vi "Basic Serial Write and Read Modified.vi"(0 "VISA resource name":refnum<visa-resource-name>="COM1", 1 "baud rate":u32=9600, 2 "data bits":u16=8 min=5 max=8 step=1, 3 "parity":u16(ring) items=["None", "Odd", "Even", "Mark", "Space"], 4 "stop bits":u16(ring)=10 items=["1.0"=10, "1.5"=15, "2.0"=20], 6 "read":bool=TRUE, 7 "flow control":u16(ring) items=["None"=0, "XON/XOFF"=1, "RTS/CTS"=2, "DTR/DSR"=4]) -> (9 "read string":string, 10 "bytes read":u32)   [LabVIEW 2016]
doc: "The Basic Serial Read and Write example performs a Serial Port Read, a Serial Port Write, or a combination of these actions. The user selects the actions (read or write) on the front panel. If both are selected, the VI will write the data first, read data, and then close the VISA session that is opened to the port. This VI will wait until the specified number of bytes is received at the port or until a termination character is read.\n\nINSTRUCTIONS:\n1) Select the serial resource and configuration parameters (baud rate, data bits, parity, stop bits, flow control).\n2) Select the operations to be performed. \n3) Connect the serial port to your device. If no device is available, perform a loopback test by doing one of the following. Short pins 2 and 3 on a RS-232 cable or short pin 4 to pin 8 and pin 5 to pin 9 on a RS-485/422 cable. \n4) Run the VI to see the data read. (The \"read string\" will match the \"string to write\" if a loopback test was performed.)\n\nNote: The parameters set for the serial port must match the parameters of the connected instrument or device. In this example, the bytes to read parameter specifies the number of bytes that the serial port reads. If there were more bytes at the port than the number specified in bytes to read, those bytes would not be read. Also, if you specify to read more bytes than the number of bytes actually read, you might receive a timeout error message.\n\nOn the block diagram, the Configure Serial Port VI sets the configuration parameters. The front panel displays the controls used to configure the basic parameters, such as baud rate, data bits, and parity. Constants configure the other parameters the user probably does not need set. After the VISA Configure Serial Port VI opens the VISA session and configures the port, the VI passes the VISA resource name to other VIs that perform operations on that VISA resource. The VISA Write function sends a command to the serial device and the VISA Read function returns data based on the command. The VISA Close function then closes the reference to the serial device. It is important to close the reference; otherwise communication through with that port through protocols other than VISA might not be possible."
uses:
  <vilib>/Instr/_visa.llb/VISA Configure Serial Port (Instr).vi
panel:
  in  "Stop":bool
  in  "Enable Termination\n Charactetr":bool
  in  "delay before read (ms)":u32=500
  # "On Windows/Linux, consider using the Instrument Driver Finder (Help>>Find Instrument Drivers) to search for an instrument driver for your instrument."
  # "Select the serial resource and the operations (Read, Write, or both) to be performed.  If both are selected, the VI will write the data first, read data and then close the VISA session that is opened to the port.  This VI will wait until the specified number of bytes is received at the port or until a termination character is read."
  # "For additional information select File >> VI Properties >> Documentation"
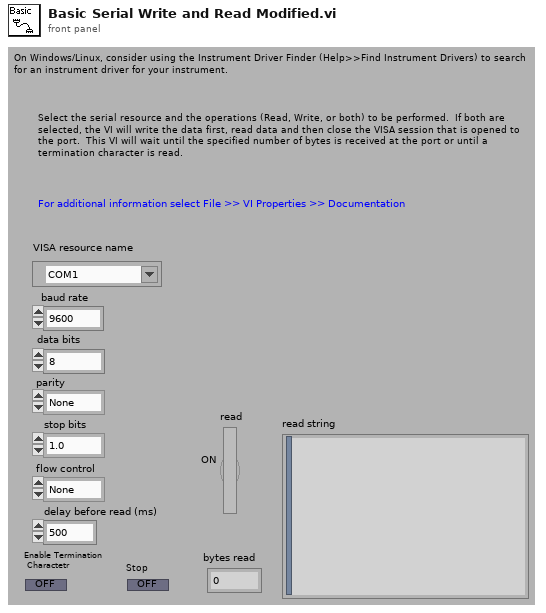
[diagram p1: front panel]
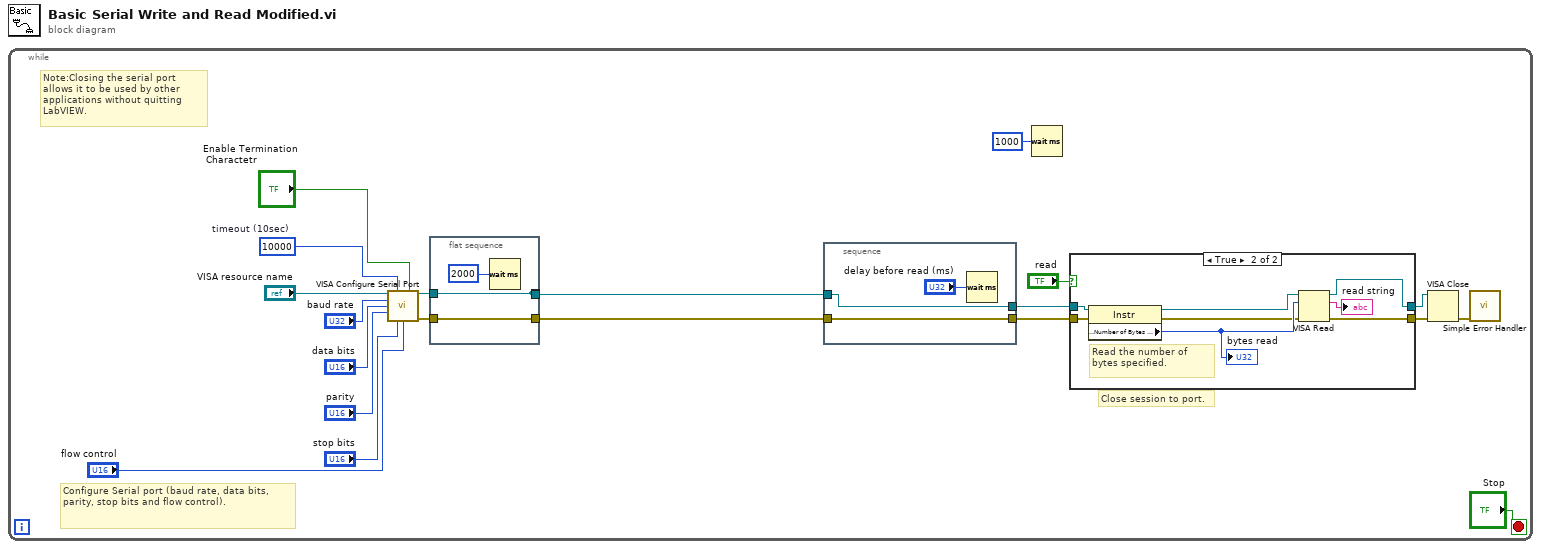
[diagram p0: block diagram]
diagram:
  n1 = while {
    stop <- "Stop" stop-if-true
    w17 = u32 10000  # timeout (10sec)
    # "Close session to port."
    # "Note:Closing the serial port allows it to be used by other applications without quitting LabVIEW."
    # "Configure Serial port (baud rate, data bits, parity, stop bits and flow control)."
    n2 = call-poly "VISA Configure Serial Port"("VISA resource name"="VISA resource name", "timeout (10sec)"=w17, "Enable Termination\nChar (T)"="Enable Termination\n Charactetr", "baud rate (9600)"="baud rate", "data bits (8)"="data bits", "parity (0:none)"="parity", "stop bits (10: 1 bit)"="stop bits", "flow control (0:none)"="flow control") -> ("VISA resource name out"=w12:refnum<visa-resource-name>, "error out"=w13:errorcluster)  [unwired: 1 in, 5 out]
    n3 = flat-sequence {
      tunnel: w13 -> [w36]
      tunnel: [w36] -> w2
      tunnel: [w34] -> _
      tunnel: w12 -> [w34]
      tunnel: [w34] -> w1
      frame #0 {
        n4 = Wait (ms)(milliseconds to wait=u32 2000) -> ()  [unwired: 1 out]
      }
    }
    n5 = stacked-sequence {
      tunnel: w1 -> [w31]
      tunnel: w2 -> [w32]
      tunnel: [w32] -> w9
      tunnel: [w31] -> w10
      frame #0 {
        n6 = Wait (ms)(milliseconds to wait="delay before read (ms)") -> ()  [unwired: 1 out]
      }
    }
    n7 = Wait (ms)(milliseconds to wait=u32 1000) -> ()  [unwired: 1 out]
    n8 = case shown="True" "read" {
      tunnel: w10 -> [w22 w30]
      tunnel: w9 -> [w21 w29]
      tunnel: [w21 w27] -> w6
      tunnel: [w22 w24] -> w7
      frame False {
      }
      frame True {
        # "Read the number of bytes specified."
        n9 = property class="Instr"(reference=w30, error in=w29) -> (reference out=w28:refnum<visa-resource-name>, error out=w25:errorcluster, "Serial Settings:Number of Bytes at Serial Port"=w26:u32)
        "bytes read" <- w26
        n10 = VISA Read(VISA resource name=w28, byte count=w26, error in (no error)=w25) -> (VISA resource name out=w24:refnum<visa-resource-name>, read buffer=→"read string":string, error out=w27:errorcluster)  [unwired: 1 out]
      }
    }
    n11 = VISA Close(VISA resource name=w7, error in (no error)=w6) -> (error out=w5:errorcluster)
    n12 = call <vilib>:"Simple Error Handler.vi"("error in (no error)"=w5) -> ()  [unwired: 1 in, 8 out]
  }
